vi "Check Overlap.vi"(8 "Cube 2":T1, 11 "Cube 1":T1) -> (2 "Full Overlap?":bool, 3 "Overlap?":bool)   [LabVIEW 2021]
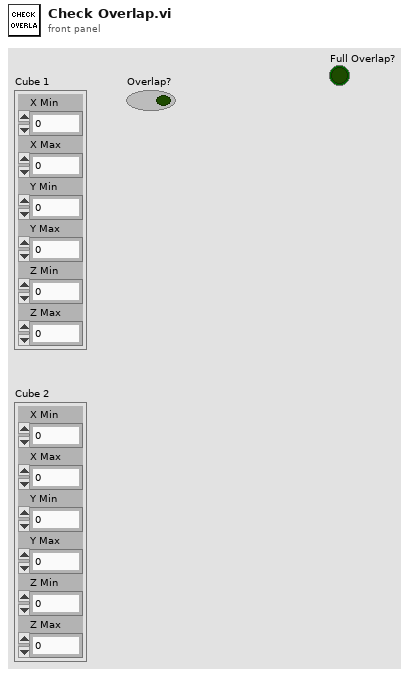
[diagram p1: front panel]
types:
  T1 = cluster{"X Min":i64, "X Max":i64, "Y Min":i64, "Y Max":i64, "Z Min":i64, "Z Max":i64}
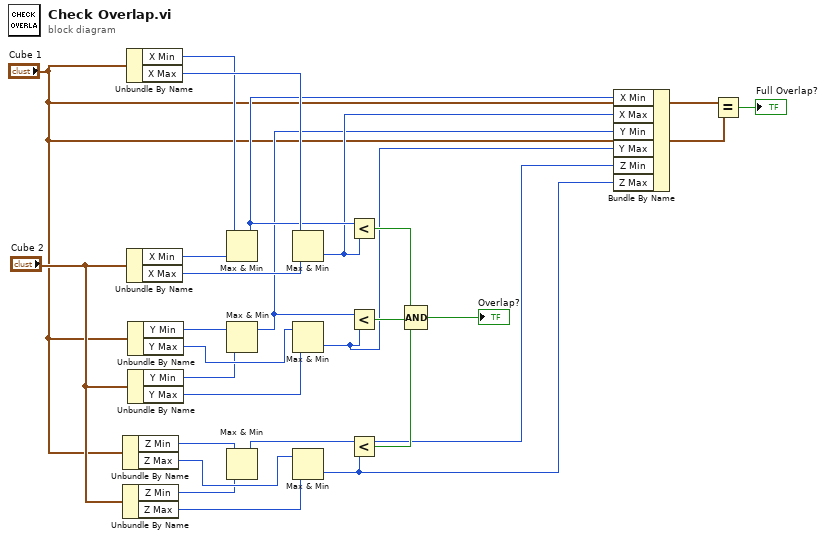
[diagram p0: block diagram]
diagram:
  n1 = Unbundle By Name("Cube 1") -> ("Z Min"=w18:i64, "Z Max"=w20:i64)
  n2 = Unbundle By Name("Cube 2") -> ("Z Min"=w19:i64, "Z Max"=w21:i64)
  n3 = Unbundle By Name("Cube 1") -> ("X Min"=w11:i64, "X Max"=w13:i64)
  n4 = Unbundle By Name("Cube 2") -> ("X Min"=w10:i64, "X Max"=w12:i64)
  n5 = Unbundle By Name("Cube 1") -> ("Y Min"=w14:i64, "Y Max"=w16:i64)
  n6 = Unbundle By Name("Cube 2") -> ("Y Min"=w15:i64, "Y Max"=w17:i64)
  n7 = Max & Min(x=w11, y=w10) -> (max(x,y)=w9:i64)  [unwired: 1 out]
  n8 = Max & Min(x=w14, y=w15) -> (max(x,y)=w7:i64)  [unwired: 1 out]
  n9 = Max & Min(x=w18, y=w19) -> (max(x,y)=w5:i64)  [unwired: 1 out]
  n10 = Max & Min(x=w13, y=w12) -> (min(x,y)=w8:i64)  [unwired: 1 out]
  n11 = Max & Min(x=w16, y=w17) -> (min(x,y)=w6:i64)  [unwired: 1 out]
  n12 = Max & Min(x=w20, y=w21) -> (min(x,y)=w4:i64)  [unwired: 1 out]
  n13 = Less?(x=w9, y=w8) -> (x < y?=w24:bool)
  n14 = Less?(x=w7, y=w6) -> (x < y?=w22:bool)
  n15 = Less?(x=w5, y=w4) -> (x < y?=w23:bool)
  n16 = Compound Arithmetic op=AND(w24, w22, w23) -> (→"Overlap?":bool)
  n17 = Bundle By Name(cluster="Cube 1", "X Min"=w9, "X Max"=w8, "Y Min"=w7, "Y Max"=w6, "Z Min"=w5, "Z Max"=w4) -> (w3:T1)
  n18 = Equal?(x="Cube 1", y=w3) -> (x = y?=→"Full Overlap?":bool)
